vi "sliderResetConnection.vi"   [LabVIEW 2017]
uses:
  globalDevices.vi
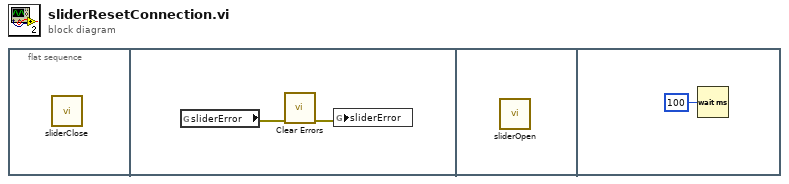
[diagram p0: block diagram]
diagram:
  n1 = flat-sequence {
    frame #0 {
      n2 = call "sliderClose.vi"() -> ()  [unwired: 2 in, 1 out]
    }
    frame #1 {
      n3 = global read "globalDevices.vi" "sliderError"() -> (w2:errorcluster)
      n4 = call <vilib>:"Clear Errors.vi"("error in (no error)"=w2) -> ("error out"=w1:errorcluster)  [unwired: 5 in, 1 out]
      n5 = global write "globalDevices.vi" "sliderError"(w1) -> ()
    }
    frame #2 {
      n6 = call "sliderOpen.vi"() -> ()  [unwired: 2 in, 1 out]
    }
    frame #3 {
      n7 = Wait (ms)(milliseconds to wait=u32 100) -> ()  [unwired: 1 out]
    }
  }
